vi "LV SciSDK SPECTRUM.vi"(7 "Spectrum Handle In":T3, 9 "Board Handle In":T1, 11 "error in (no error)":errorcluster) -> (4 "NI Error Code":i32, 6 "Spectrum Buffer Out":T2, 8 "Spectrum Handle Out":T3, 10 "Board Handle Out":T1, 15 "error out":errorcluster)   [LabVIEW 2021, in "SciSDK_Labview.lvlib"]
doc: "You need this VI to read data from a spectrum component"
uses:
  SciSDK_Labview.lvlib
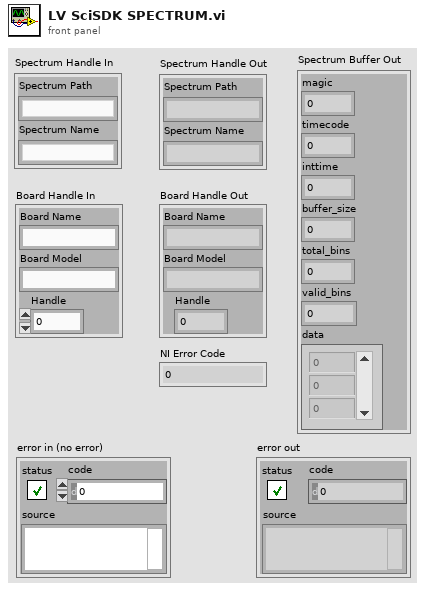
[diagram p1: front panel]
types:
  T1 = cluster{"Board Name":string, "Board Model":string, "Handle":u64}
  T2 = cluster{"magic":u32, "timecode":u32, "inttime":u32, "buffer_size":u32, "total_bins":u32, "valid_bins":u32, "data":i32[]}
  T3 = cluster{"Spectrum Path":string, "Spectrum Name":string}
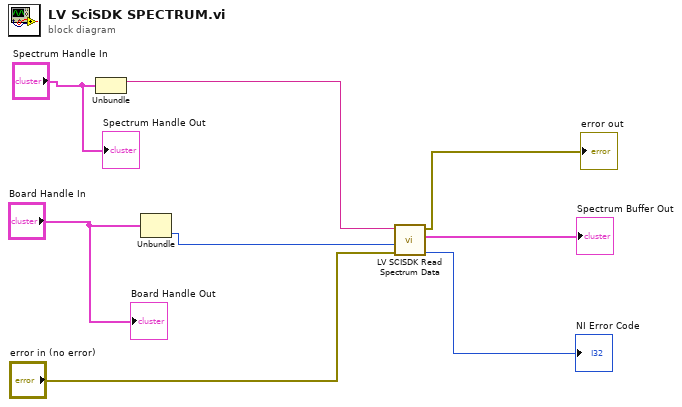
[diagram p0: block diagram]
diagram:
  n1 = Unbundle("Spectrum Handle In") -> ("Spectrum Path"=w5:string)  [unwired: 1 out]
  n2 = Unbundle("Board Handle In") -> ("Handle"=w3:u64)  [unwired: 2 out]
  n3 = call "LV SCISDK Read Spectrum Data.vi"("Path 2"=w5, "handle 2"=w3, "error in (no error) 2"="error in (no error)") -> ("error out 2"=→"error out":errorcluster, "buffer out"=→"Spectrum Buffer Out":T2, "function return 2"=→"NI Error Code":i32)  [unwired: 4 in, 1 out]
  "Spectrum Handle Out" <- "Spectrum Handle In"
  "Board Handle Out" <- "Board Handle In"
